vi "tree study.vi"() -> ()   [LabVIEW 2015]
panel:
  in  "Tree":string(tree)
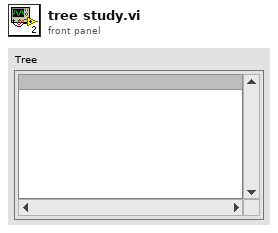
[diagram p1: front panel]
types:
  T1 = cluster{"Left Cell String":string, "Child Text":string[], "Child Tag":string, "Item Indent":i32, "Child Only?":bool, "Glyph Index":i32}[]
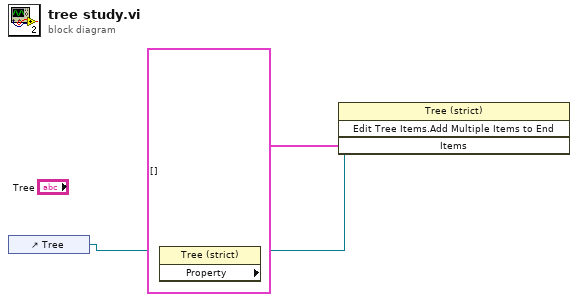
[diagram p0: block diagram]
diagram:
  n1 = control-ref of="Tree"() -> (w2:refnum<vi>)
  n2 = property class="Tree (strict)" props=[](reference=w2) -> ()  [unwired: 1 in, 3 out]
  n3 = invoke class="Tree (strict)" method="Edit Tree Items.Add Multiple Items to End"(reference=w2, "Items"=T1 []) -> ()  [unwired: 2 in, 4 out]
